vi "設定品番選択画面.vi"() -> (20 "品番設定_品番品名":T1)   [LabVIEW 2021]
uses:
  <vilib>/Utility/config.llb/Read Key (String).vi
  <vilib>/Utility/config.llb/NI_LVConfig.lvlib
panel:
  out "エラー出力 2":errorcluster caption="エラー出力"
  out "error in (no error) 4":errorcluster caption="エラー入力（エラーなし）"
  in  "ini error in (no error)":errorcluster caption="エラー入力（エラーなし）"
  out "iniフォルダパス取得":path
  in  "品番5":bool
  out "エラー出力":errorcluster
  in  "品番8":bool
  in  "品番7":bool
  in  "品番6":bool
  in  "品番4":bool
  in  "品番3":bool
  in  "品番2":bool
  in  "品番1":bool
  in  "TOPへ戻る":bool
  # "設定する品番を選択"
  # "-"
  # "品番"
  # "品名"
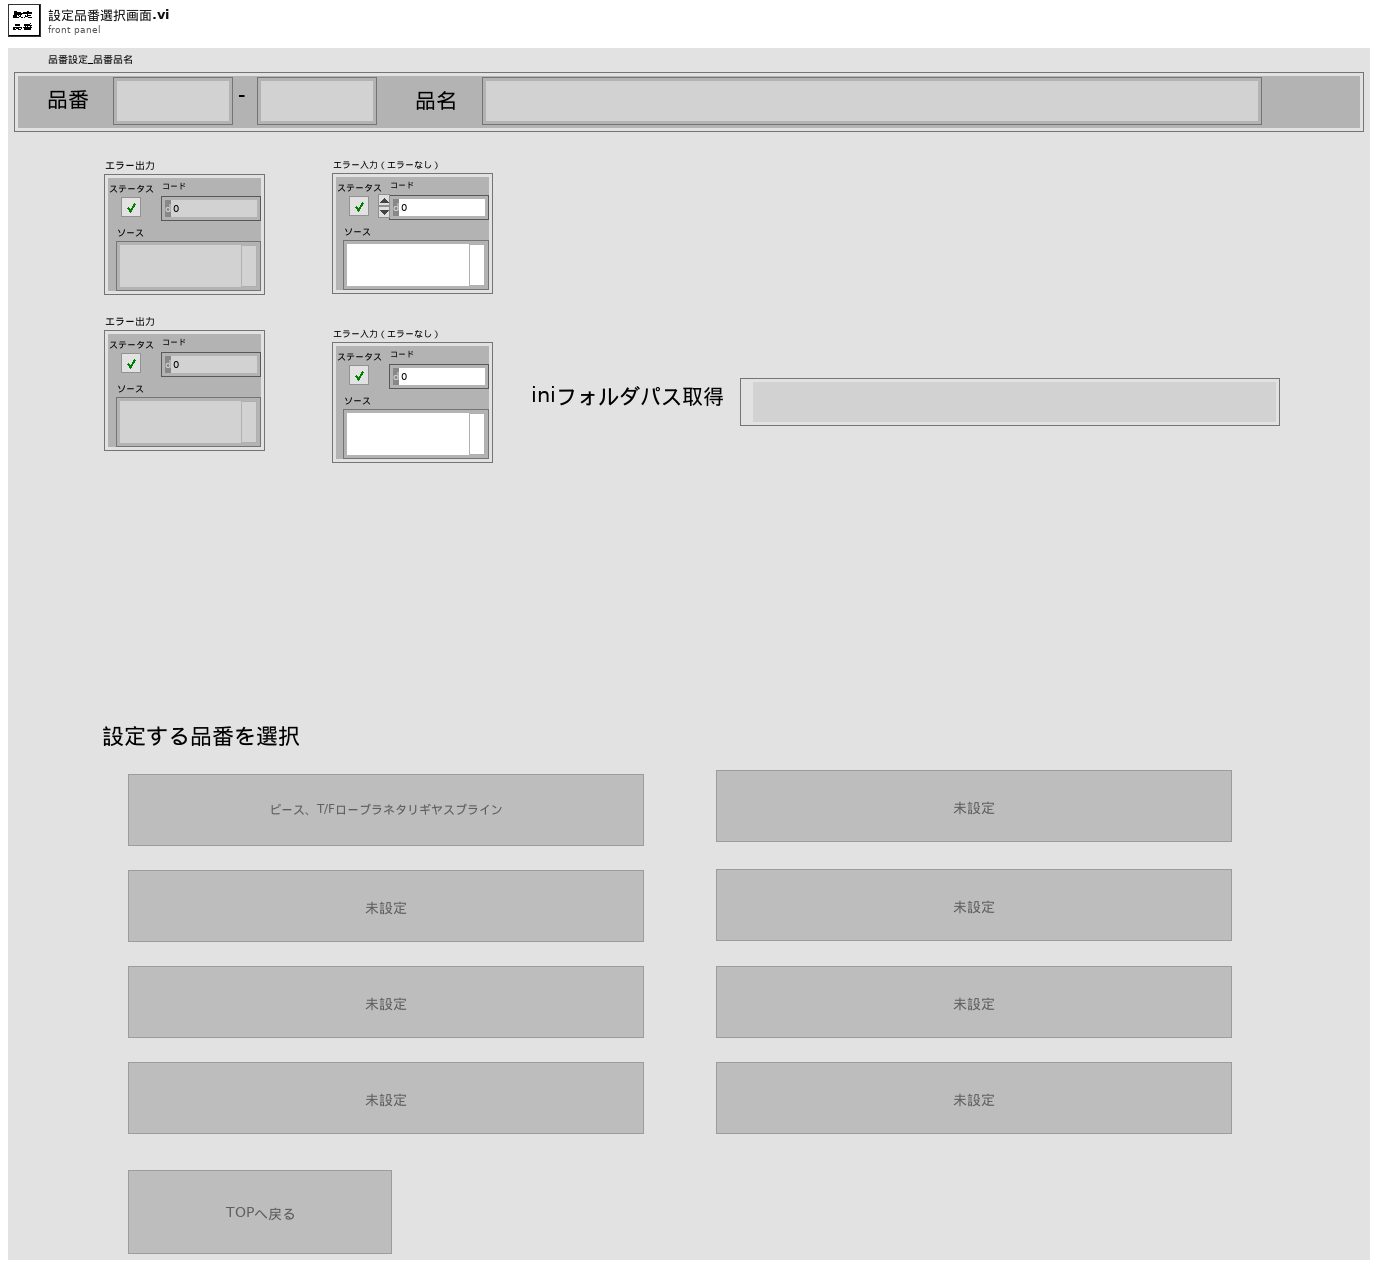
[diagram p1: front panel]
types:
  T1 = typedef "品番・品名選択用.ctl" = cluster{"品名":string, "品番前":string, "品番後":string}
  T2 = enum8{"Enabled", "Disabled", "Disabled and Grayed Out"}
  T3 = typedef "NI_LVConfig.lvlib/Config Data RefNum.ctl" = refnum<k1>
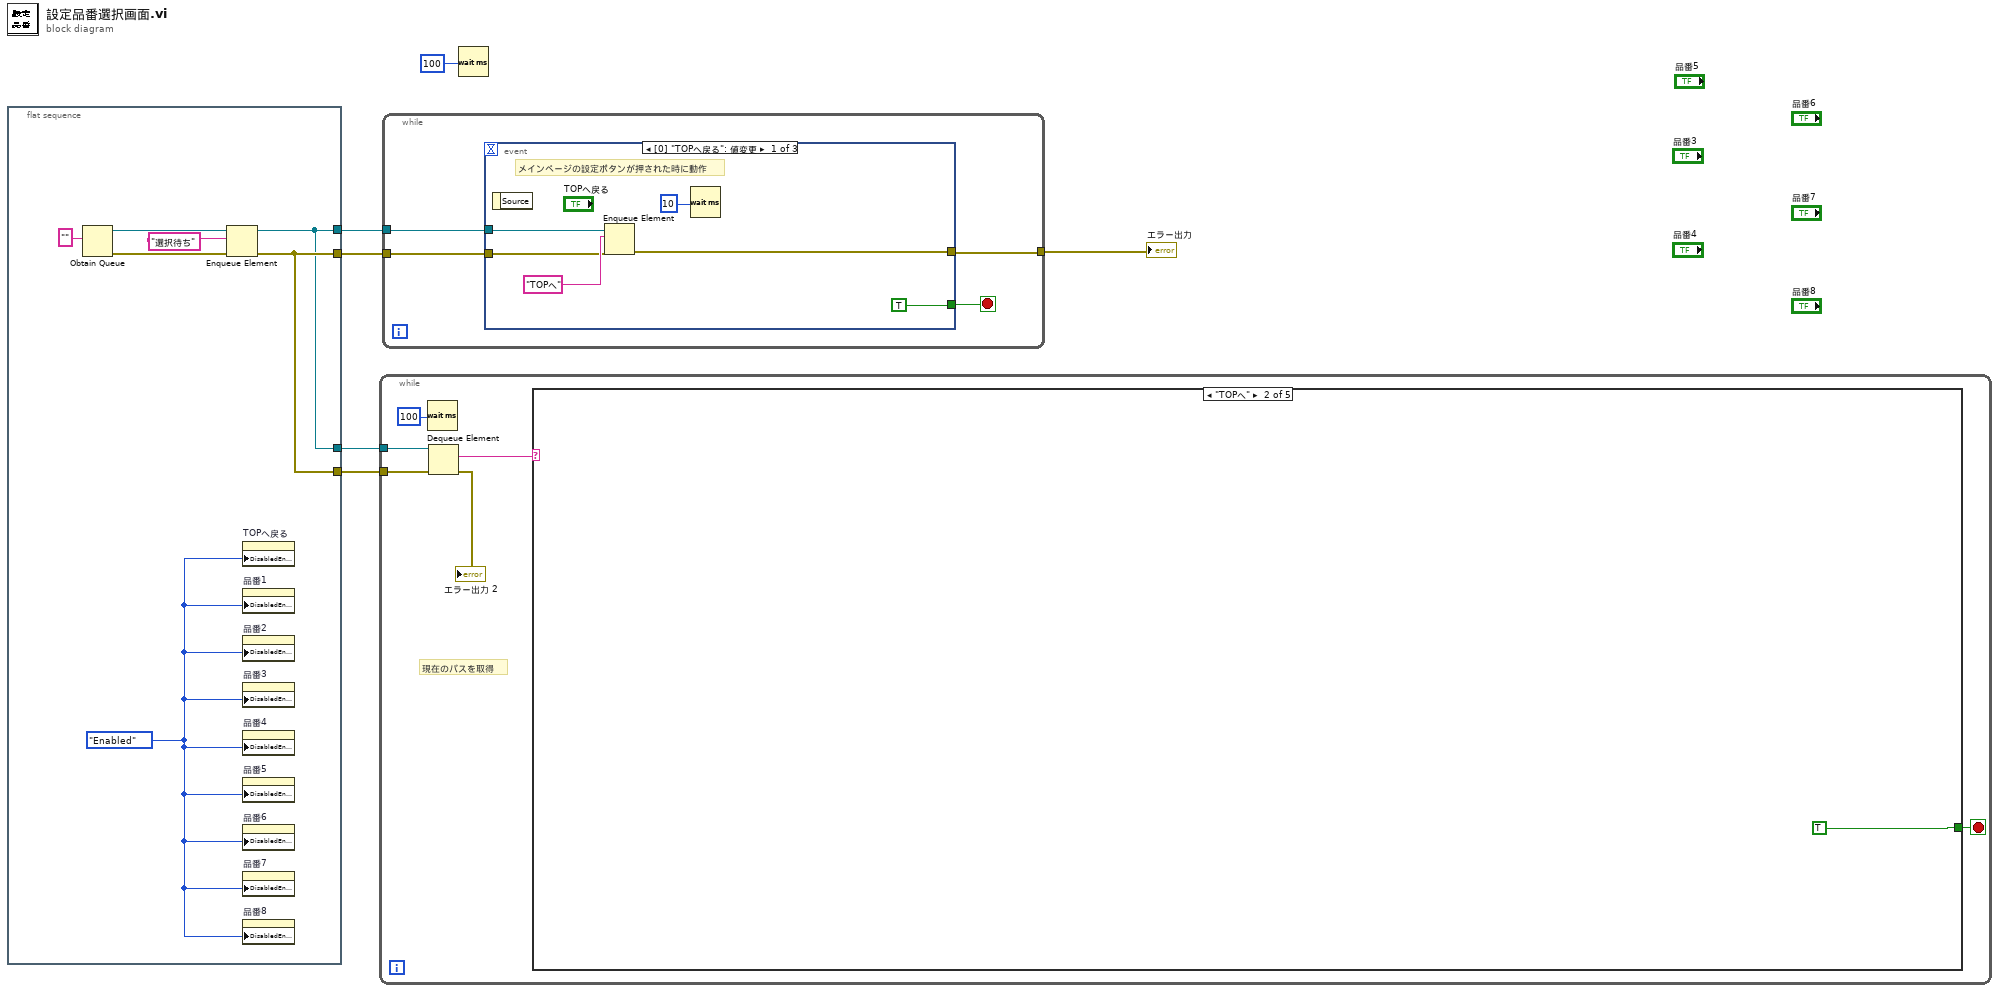
[diagram p0: block diagram]
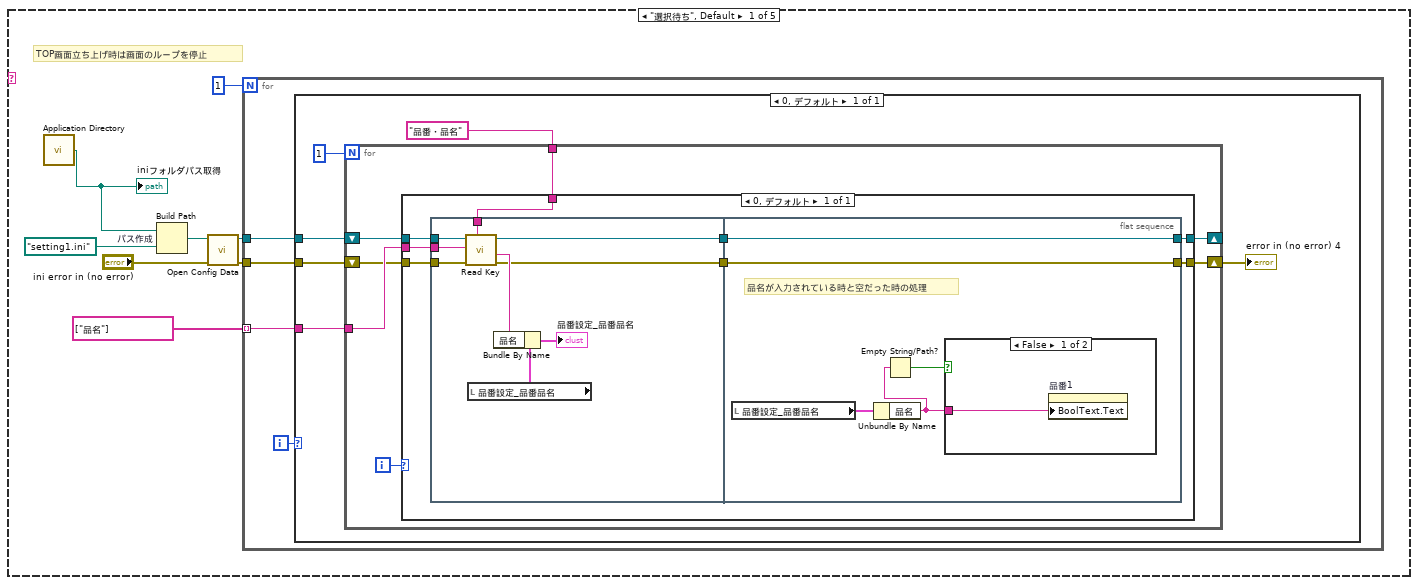
[diagram p2: hidden frame]
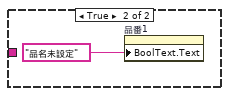
[diagram p3: hidden frame]
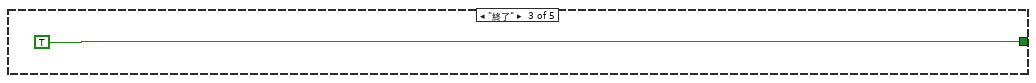
[diagram p4: hidden frame]
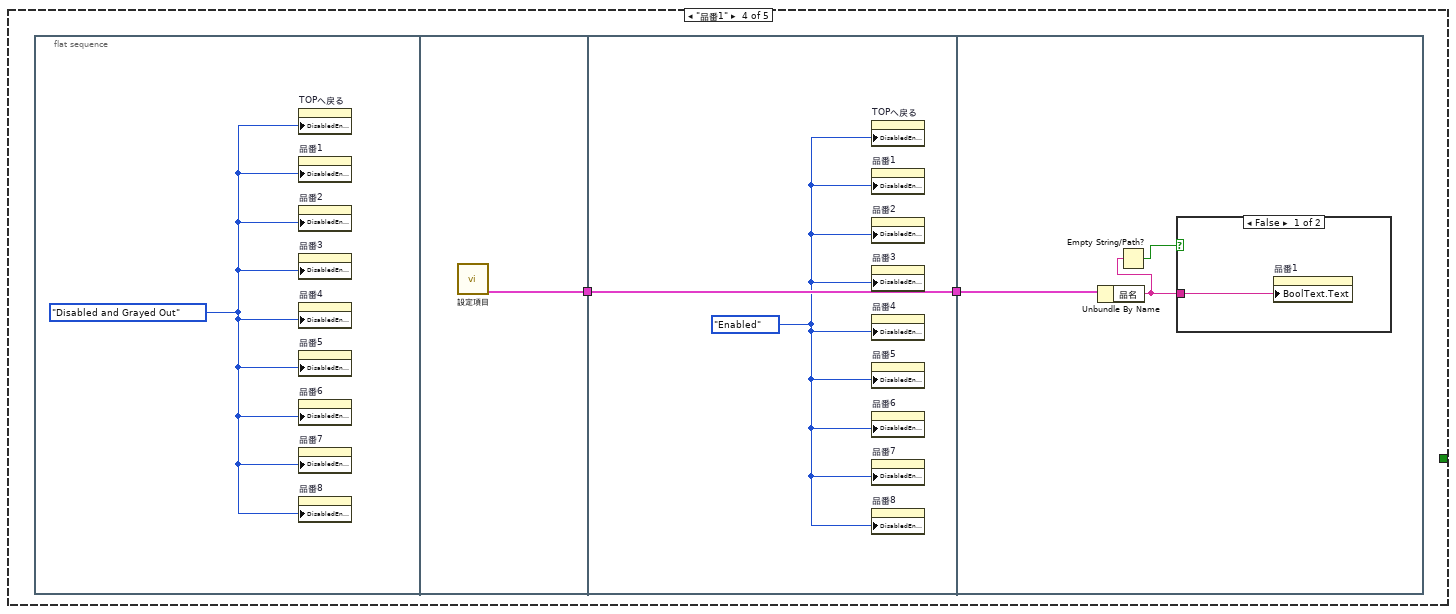
[diagram p5: hidden frame]
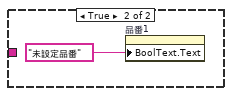
[diagram p6: hidden frame]
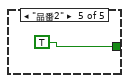
[diagram p7: hidden frame]
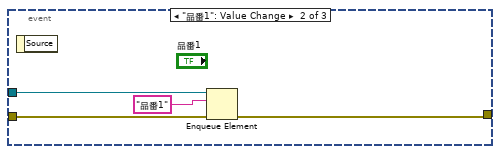
[diagram p8: hidden frame]
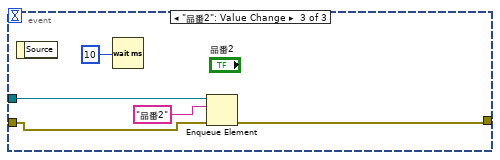
[diagram p9: hidden frame]
diagram:
  n1 = flat-sequence {
    tunnel: [w9] -> w5
    tunnel: [w8] -> w4
    tunnel: [w9] -> w3
    tunnel: [w8] -> w2
    frame #0 {
      w7 = T2."Enabled" ("無効")
      n2 = Obtain Queue(element data type="") -> (queue out=w12:refnum<queue>, error out=w10:errorcluster)  [unwired: 4 in, 1 out]
      n3 = Enqueue Element(queue=w12, element="選択待ち", error in (no error)=w10) -> (queue out=w8:refnum<queue>, error out=w9:errorcluster)  [unwired: 1 in, 1 out]
      n4 = property on="TOPへ戻る" class="Bool"("DisabledEnum"=w7) -> ()  [unwired: 2 in, 2 out]
      n5 = property on="品番1" class="Bool"("DisabledEnum"=w7) -> ()  [unwired: 2 in, 2 out]
      n6 = property on="品番2" class="Bool"("DisabledEnum"=w7) -> ()  [unwired: 2 in, 2 out]
      n7 = property on="品番3" class="Bool"("DisabledEnum"=w7) -> ()  [unwired: 2 in, 2 out]
      n8 = property on="品番4" class="Bool"("DisabledEnum"=w7) -> ()  [unwired: 2 in, 2 out]
      n9 = property on="品番5" class="Bool"("DisabledEnum"=w7) -> ()  [unwired: 2 in, 2 out]
      n10 = property on="品番6" class="Bool"("DisabledEnum"=w7) -> ()  [unwired: 2 in, 2 out]
      n11 = property on="品番7" class="Bool"("DisabledEnum"=w7) -> ()  [unwired: 2 in, 2 out]
      n12 = property on="品番8" class="Bool"("DisabledEnum"=w7) -> ()  [unwired: 2 in, 2 out]
    }
  }
  n13 = while {
    tunnel: w3 -> [w15]
    tunnel: w2 -> [w14]
    stop <- w19 stop-if-true
    # "現在のパスを取得"
    n14 = Wait (ms)(milliseconds to wait=100) -> ()  [unwired: 1 out]
    n15 = Dequeue Element(queue=w14, error in (no error)=w15) -> (element=w16:string, error out=→"エラー出力 2":errorcluster)  [unwired: 1 in, 2 out]
    n16 = case shown="\"TOPへ\"" w16 {
      tunnel: [_ TRUE TRUE _ TRUE] -> w19
      frame "選択待ち", Default {
        # "TOP画面立ち上げ時は画面のループを停止"
        n17 = call <vilib>:"Application Directory.vi"() -> ("Application Directory"=w20:path)
        "iniフォルダパス取得" <- w20
        n18 = Build Path "パス作成"(base path=w20, name or relative path=path "setting1.ini") -> (appended path=w26:path)
        n19 = call <vilib>:"Open Config Data.vi"("error in (no error)"="ini error in (no error)", "configuration file path"=w26) -> ("error out"=w21:errorcluster, "refnum"=w22:T3)  [unwired: 1 in, 7 out]
        n20 = for {
          N: 1 -> [_]
          tunnel: string[] ["品名"] -> [w30] mode=indexing
          tunnel: w22 -> [w29]
          tunnel: w21 -> [w28]
          i -> [w31]
          n21 = case shown="0, デフォルト" w31 {
            tunnel: w30 -> [w34]
            tunnel: w29 -> [w33]
            tunnel: w28 -> [w32]
            frame 0, Default {
              n22 = for {
                N: 1 -> [_]
                shift-right: [w42] -> _
                shift-left: w33 -> [w43]
                tunnel: w34 -> [w41]
                tunnel: "品番・品名" -> [w40]
                shift-right: [w38] -> w35
                shift-left: w32 -> [w39]
                i -> [w44]
                n23 = case shown="0, デフォルト" w44 {
                  tunnel: w43 -> [w51]
                  tunnel: [w47] -> w42
                  tunnel: w41 -> [w50]
                  tunnel: w40 -> [w52]
                  tunnel: w39 -> [w49]
                  tunnel: [w48] -> w38
                  frame 0, Default {
                    n24 = flat-sequence {
                      tunnel: w52 -> [w58]
                      tunnel: w51 -> [w57]
                      tunnel: w50 -> [w56]
                      tunnel: w49 -> [w55]
                      tunnel: [w54] -> w46
                      tunnel: [w53] -> w45
                      tunnel: [w65] -> w47
                      tunnel: [w66] -> w48
                      tunnel: w46 -> [w66]
                      tunnel: w45 -> [w65]
                      frame #0 {
                        n25 = call-poly <vilib>:"Read Key.vi"("section"=w58, "error in (no error)"=w55, "key"=w56, "refnum"=w57) -> ("error out"=w54:errorcluster, "value"=w60:string, "refnum out"=w53:T3)  [unwired: 4 in, 1 out]
                        n26 = local read "品番設定_品番品名"() -> (w61:T1)
                        n27 = Bundle By Name(cluster=w61, "品名"=w60) -> (→"品番設定_品番品名":T1)
                      }
                      frame #1 {
                        # "品名が入力されている時と空だった時の処理"
                        n28 = local read "品番設定_品番品名"() -> (w63:T1)
                        n29 = Unbundle By Name(w63) -> ("品名"=w62:string)
                        n30 = Empty String/Path?(string/path=w62) -> (empty?=w64:bool)
                        n31 = case shown="FALSE" w64 {
                          tunnel: w62 -> [w67 _]
                          frame False {
                            n32 = property on="品番1" class="Bool"("BoolText.Text"=w67) -> ()  [unwired: 2 in, 2 out]
                          }
                          frame True {
                            n33 = property on="品番1" class="Bool"("BoolText.Text"="品名未設定") -> ()  [unwired: 2 in, 2 out]
                          }
                        }
                      }
                    }
                  }
                }
              }
              "error in (no error) 4" <- w35
            }
          }
        }
      }
      frame "TOPへ" {
      }
      frame "終了" {
      }
      frame "品番1" {
        n34 = flat-sequence {
          tunnel: [w74] -> w71
          tunnel: [w76] -> w72
          tunnel: w71 -> [w76]
          tunnel: w72 -> [w77]
          frame #0 {
            w73 = T2."Disabled and Grayed Out" ("無効")
            n35 = property on="TOPへ戻る" class="Bool"("DisabledEnum"=w73) -> ()  [unwired: 2 in, 2 out]
            n36 = property on="品番1" class="Bool"("DisabledEnum"=w73) -> ()  [unwired: 2 in, 2 out]
            n37 = property on="品番2" class="Bool"("DisabledEnum"=w73) -> ()  [unwired: 2 in, 2 out]
            n38 = property on="品番3" class="Bool"("DisabledEnum"=w73) -> ()  [unwired: 2 in, 2 out]
            n39 = property on="品番4" class="Bool"("DisabledEnum"=w73) -> ()  [unwired: 2 in, 2 out]
            n40 = property on="品番5" class="Bool"("DisabledEnum"=w73) -> ()  [unwired: 2 in, 2 out]
            n41 = property on="品番6" class="Bool"("DisabledEnum"=w73) -> ()  [unwired: 2 in, 2 out]
            n42 = property on="品番7" class="Bool"("DisabledEnum"=w73) -> ()  [unwired: 2 in, 2 out]
            n43 = property on="品番8" class="Bool"("DisabledEnum"=w73) -> ()  [unwired: 2 in, 2 out]
          }
          frame #1 {
            n44 = call "設定項目.vi"() -> ("品番・品名クラスタ_設定 _表示器"=w74:T1)  [unwired: 15 in]
          }
          frame #2 {
            w75 = T2."Enabled" ("無効")
            n45 = property on="TOPへ戻る" class="Bool"("DisabledEnum"=w75) -> ()  [unwired: 2 in, 2 out]
            n46 = property on="品番1" class="Bool"("DisabledEnum"=w75) -> ()  [unwired: 2 in, 2 out]
            n47 = property on="品番2" class="Bool"("DisabledEnum"=w75) -> ()  [unwired: 2 in, 2 out]
            n48 = property on="品番3" class="Bool"("DisabledEnum"=w75) -> ()  [unwired: 2 in, 2 out]
            n49 = property on="品番4" class="Bool"("DisabledEnum"=w75) -> ()  [unwired: 2 in, 2 out]
            n50 = property on="品番5" class="Bool"("DisabledEnum"=w75) -> ()  [unwired: 2 in, 2 out]
            n51 = property on="品番6" class="Bool"("DisabledEnum"=w75) -> ()  [unwired: 2 in, 2 out]
            n52 = property on="品番7" class="Bool"("DisabledEnum"=w75) -> ()  [unwired: 2 in, 2 out]
            n53 = property on="品番8" class="Bool"("DisabledEnum"=w75) -> ()  [unwired: 2 in, 2 out]
          }
          frame #3 {
            n54 = Unbundle By Name(w77) -> ("品名"=w79:string)
            n55 = Empty String/Path?(string/path=w79) -> (empty?=w78:bool)
            n56 = case shown="FALSE" w78 {
              tunnel: w79 -> [w80 _]
              frame False {
                n57 = property on="品番1" class="Bool"("BoolText.Text"=w80) -> ()  [unwired: 2 in, 2 out]
              }
              frame True {
                n58 = property on="品番1" class="Bool"("BoolText.Text"="未設定品番") -> ()  [unwired: 2 in, 2 out]
              }
            }
          }
        }
      }
      frame "品番2" {
      }
    }
  }
  n59 = while {
    tunnel: w4 -> [w86]
    tunnel: w5 -> [w84]
    tunnel: [w83] -> w1
    stop <- w85 stop-if-true
    n60 = event shown="[0] \"TOPへ戻る\": 値変更" {
      selector: _ -> [_ _ _]
      dyn-events: _ -> [_ _ _]
      timeout: _ -> [_ _ _]
      tunnel: w86 -> [w92 w95 w100]
      tunnel: [TRUE _ _] -> w85
      tunnel: w84 -> [w90 w94 w99]
      tunnel: [w89 w93 w98] -> w83
      event "TOPへ戻る": Value Change {
        # "メインページの設定ボタンが押された時に動作"
        n61 = event-data() -> ()  [unwired: 1 in, 1 out]
        n62 = Enqueue Element(queue=w92, element="TOPへ", error in (no error)=w90) -> (error out=w89:errorcluster)  [unwired: 1 in, 2 out]
        n63 = Wait (ms)(milliseconds to wait=10) -> ()  [unwired: 1 out]
      }
      event "品番1": Value Change {
        n64 = event-data() -> ()  [unwired: 1 in, 1 out]
        n65 = Enqueue Element(queue=w95, element="品番1", error in (no error)=w94) -> (error out=w93:errorcluster)  [unwired: 1 in, 2 out]
      }
      event "品番2": Value Change {
        n66 = event-data() -> ()  [unwired: 1 in, 1 out]
        n67 = Wait (ms)(milliseconds to wait=10) -> ()  [unwired: 1 out]
        n68 = Enqueue Element(queue=w100, element="品番2", error in (no error)=w99) -> (error out=w98:errorcluster)  [unwired: 1 in, 2 out]
      }
    }
  }
  "エラー出力" <- w1
  n69 = Wait (ms)(milliseconds to wait=100) -> ()  [unwired: 1 out]
